vi "AR-DO-write.vi"(8 "error in (no error)":errorcluster, 10 "Data":bool[](array[boolean]), 11 "DO task in":refnum<k21>) -> (0 "error out":errorcluster, 3 "DO task out":refnum<k21>)   [LabVIEW 2021]
uses:
  <vilib>/DAQmx/write.llb/DAQmx Write (Digital 1D Bool 1Chan 1Samp).vi
  <vilib>/DAQmx/miscellaneous.llb/DAQmx Fill In Error Info.vi
  <resource>/objmgr/daqmx.rc
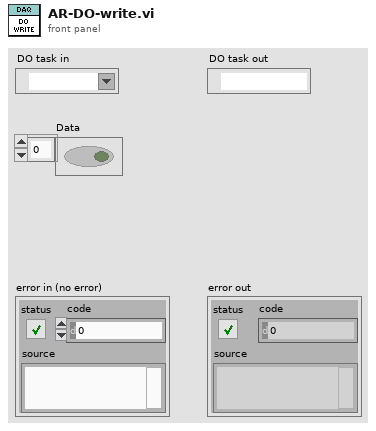
[diagram p1: front panel]
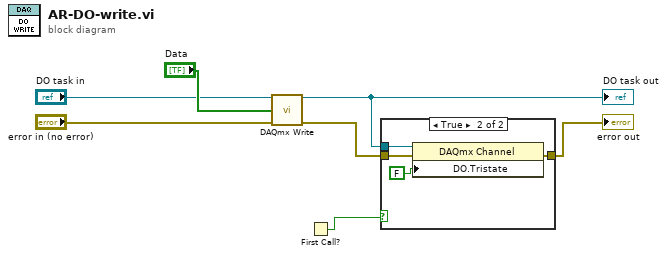
[diagram p0: block diagram]
diagram:
  n1 = call-poly <vilib>:"DAQmx Write.vi"("task/channels in"="DO task in", "data"="Data", "error in"="error in (no error)") -> ("task out"=w5:refnum<k21>, "error out"=w6:errorcluster)  [unwired: 10 in, 1 out]
  "DO task out" <- w5
  n2 = First Call?() -> (First Call?: T/F=w1:bool)
  n3 = case shown="True" w1 {
    tunnel: w5 -> [_ w11]
    tunnel: w6 -> [w8 w10]
    tunnel: [w8 w9] -> w7
    frame False {
    }
    frame True {
      n4 = property class="DAQmx Channel"(reference=w11, error in=w10, "DO.Tristate"=FALSE) -> (error out=w9:errorcluster)  [unwired: 1 out]
    }
  }
  "error out" <- w7
